vi "Floc Interface.vi"(8 "error in":errorcluster, 9 "ROI":T3, 10 "Interface inputs":T1={"Elevation of top of Field of View (cm)"=10.0, "Field of View Height (cm)"=-0.1, "Smooth Length (cm)"=5.0, "Min derivative magnitude"=5.0, "Color Plane"=enum."Green"} {"Smooth Length (cm)" min=0.01 max=1000.0 step=0.1; "Field of View Height (cm)" min=0.1 max=1000.0 step=0.1}, 11 "Image":T2) -> (0 "error out":errorcluster, 1 "max value":dbl, 2 "Interface elevation":dbl, 4 "min value":dbl)   [LabVIEW 2015, in "Camera SubVIs.lvlib"]
uses:
  Camera SubVIs.lvlib
  <vilib>/vision/Image Controls.llb/IMAQ Image.ctl
  Interface Inputs.ctl
  <vilib>/Analysis/baseanly.llb/Mean (DBL).vi
  <vilib>/Analysis/NI_AALBase.lvlib
  <vilib>/Analysis/NI_AALPro.lvlib
  <vilib>/vision/NI_Vision_Development_Module.lvlib
  <resource>/objmgr/IMAQImage.rc
panel:
  out "error out 2":errorcluster
  out "ROI Out":T2(plugin-control)
  out "min index":i32
  out "max index":i32
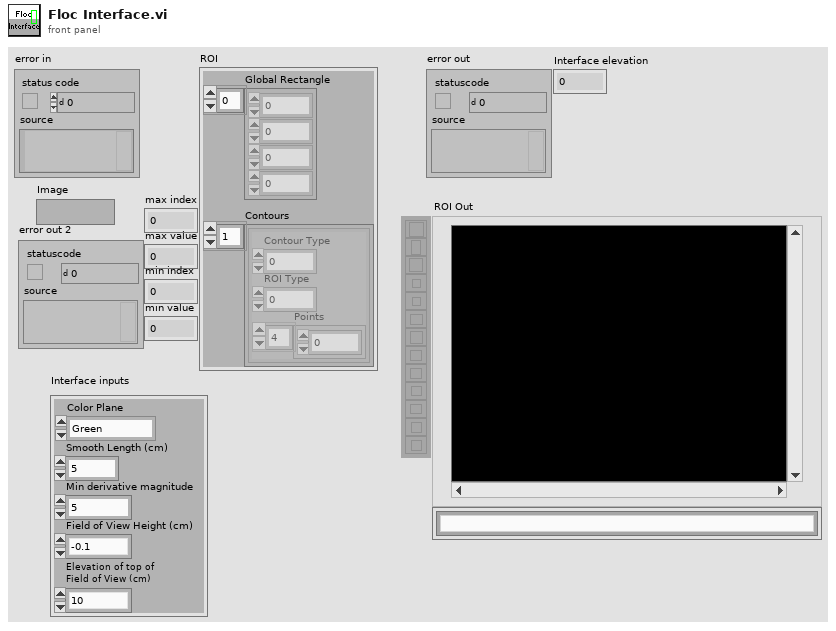
[diagram p1: front panel]
types:
  T1 = typedef "Camera SubVIs.lvlib/Interface Inputs.ctl" = cluster{"Elevation of top of Field of View (cm)":dbl, "Field of View Height (cm)":dbl, "Smooth Length (cm)":dbl, "Min derivative magnitude":dbl, "Color Plane":enum16{"Red", "Green", "Blue", "Combined"}}
  T2 = typedef "IMAQ Image.ctl" = refnum<image>
  T3 = cluster{"Global Rectangle":i32[], "Contours":cluster{"Contour Type":u32, "ROI Type":u32, "Points":i32[]}[]}
  T4 = typedef "Image Type" = u32
  T5 = cluster{"Global Rectangle[0]":i32, "Global Rectangle[1]":i32, "Global Rectangle[2]":i32, "Global Rectangle[3]":i32}
  T6 = cluster{"Red (or Hue) value":u8, "Green (or Sat) value":u8, "Blue (or Light or Val) value":u8}[][]
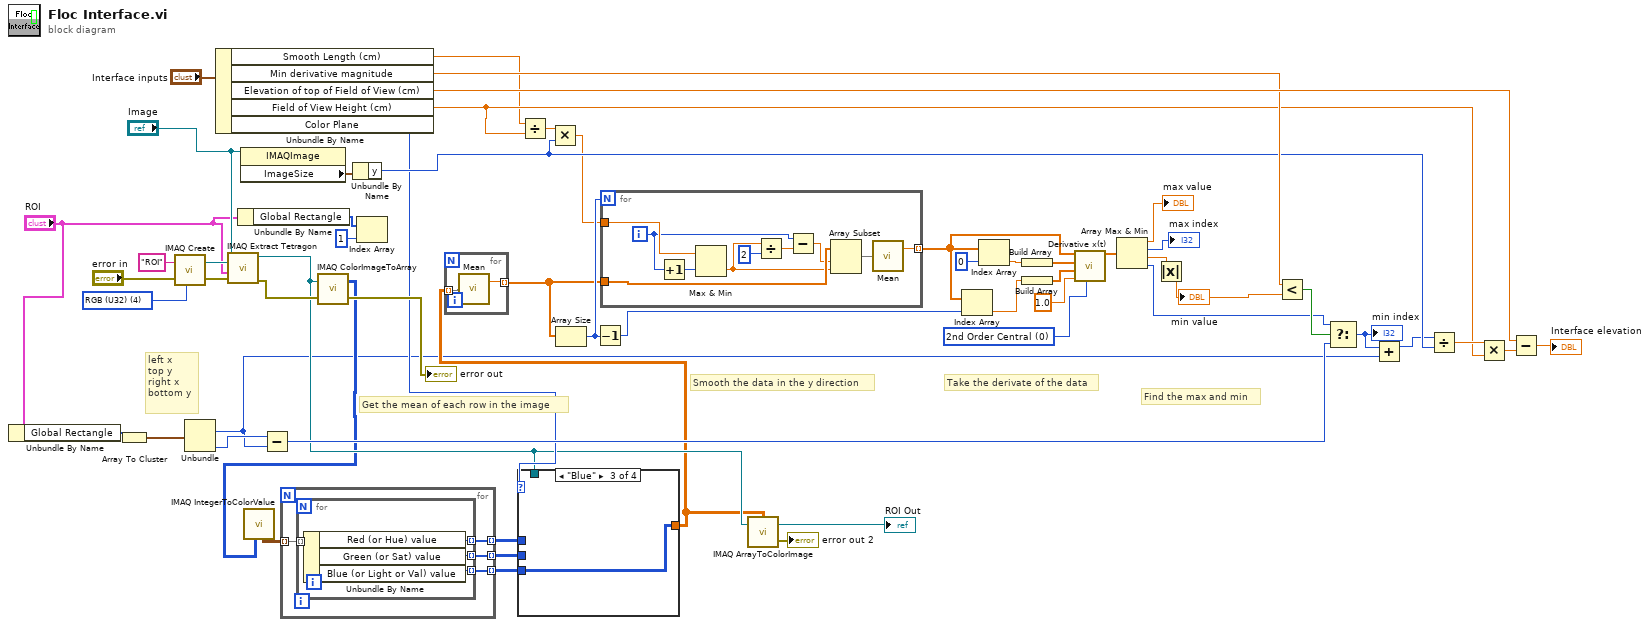
[diagram p0: block diagram]
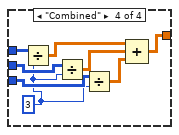
[diagram p4: hidden frame]
diagram:
  w43 = T4 4 items=["Grayscale (U8)", "Grayscale (I16)", "Grayscale (SGL)", "Complex (CSG)", "RGB (U32)", "HSL (U32)", "RGB (U64)", "Grayscale (U16)"] ("Image Type")
  w45 = u16 0 items=["2nd Order Central", "4th Order Central", "Forward", "Backward"] ("method")
  # "left x\ntop y\nright x\nbottom y"
  # "Find the max and min"
  # "Take the derivate of the data"
  # "Smooth the data in the y direction"
  # "Get the mean of each row in the image"
  n1 = Unbundle By Name("ROI") -> ("Global Rectangle"=w35:i32[])
  n2 = Array To Cluster(array=w35) -> (cluster=w34:T5)
  n3 = call "IMAQ Create"("Image Name"="ROI", "Image Type"=w43, "error in (no error)"="error in") -> ("New Image"=w40:T2, "error out"=w41:errorcluster)  [unwired: 1 in, 1 out]
  n4 = Unbundle(w34) -> ("Global Rectangle[1]"=w1:i32, "Global Rectangle[3]"=w33:i32)  [unwired: 2 out]
  n5 = Unbundle By Name("Interface inputs") -> ("Smooth Length (cm)"=w22:dbl, "Min derivative magnitude"=w25:dbl, "Elevation of top of Field of View (cm)"=w27:dbl, "Field of View Height (cm)"=w23:dbl, "Color Plane"=w17:enum16{"Red", "Green", "Blue", "Combined"})
  n6 = call-poly "IMAQ Extract Tetragon"("error in (no error)"=w41, "ROI Descriptor"="ROI", "Image Dst"=w40, "Image Src"="Image") -> ("error out"=w18:errorcluster, "Image Dst Out"=w14:T2)  [unwired: 6 in]
  n7 = Unbundle By Name("ROI") -> ("Global Rectangle"=w4:i32[])
  n8 = property class="IMAQImage"(reference="Image") -> ("ImageSize"=w6:cluster{"x":i32, "y":i32})  [unwired: 1 in, 2 out]
  n9 = Subtract(x=w33, y=w1) -> (x-y=w32:i32)
  n10 = call "IMAQ ColorImageToArray"("Image"=w14, "error in (no error)"=w18) -> ("Image Pixels (U32)"=w9:u32[][], "error out"=→"error out":errorcluster)  [unwired: 2 in, 1 out]
  n11 = call "IMAQ IntegerToColorValue"("2D U32 array"=w9) -> ("2D Color value array"=w13:T6)  [unwired: 4 in, 3 out]
  n12 = for {
    tunnel: w13 -> [w62] mode=indexing
    tunnel: [w61] -> w12 mode=indexing
    tunnel: [w60] -> w11 mode=indexing
    tunnel: [w59] -> w10 mode=indexing
    n13 = for {
      tunnel: w62 -> [w66] mode=indexing
      tunnel: [w65] -> w61 mode=indexing
      tunnel: [w64] -> w60 mode=indexing
      tunnel: [w63] -> w59 mode=indexing
      n14 = Unbundle By Name(w66) -> ("Red (or Hue) value"=w65:u8, "Green (or Sat) value"=w64:u8, "Blue (or Light or Val) value"=w63:u8)
    }
  }
  n15 = Unbundle By Name(w6) -> ("y"=w20:i32)
  n16 = Index Array(array=w4, index=1) -> ()  [unwired: 1 out]
  n17 = case shown="\"Blue\"" w17 {
    tunnel: [w67 w68 w69 w70] -> w8
    tunnel: w14 -> [_ _ _ _]
    tunnel: w12 -> [w67 _ _ w77]
    tunnel: w11 -> [_ w68 _ w76]
    tunnel: w10 -> [_ _ w69 w75]
    frame "Red", Default {
    }
    frame "Green" {
    }
    frame "Blue" {
    }
    frame "Combined" {
      w74 = 3
      n18 = Divide(x=w77, y=w74) -> (x/y=w73:dbl[][])
      n19 = Divide(x=w76, y=w74) -> (x/y=w72:dbl[][])
      n20 = Divide(x=w75, y=w74) -> (x/y=w71:dbl[][])
      n21 = Compound Arithmetic op=ADD(w73, w72, w71) -> (w70:dbl[][])
    }
  }
  n22 = for {
    tunnel: w8 -> [w79] mode=indexing
    tunnel: [w78] -> w7 mode=indexing
    n23 = call-poly <vilib>:"Mean.vi"("X"=w79) -> ("mean"=w78:dbl)  [unwired: 1 out]
  }
  n24 = Divide(x=w22, y=w23) -> (x/y=w21:dbl)
  n25 = Multiply(x=w21, y=w20) -> (x*y=w19:dbl)
  n26 = Array Size(array=w7) -> (size(s)=w52:i32)
  n27 = Decrement(x=w52) -> (x-1=w49:i32)
  n28 = for {
    N: w52 -> [_]
    tunnel: w7 -> [w89]
    tunnel: w19 -> [w86]
    tunnel: [w87] -> w51 mode=indexing
    i -> [w82]
    n29 = Increment(x=w82) -> (x+1=w85:i32)
    n30 = Max & Min(x=w86, y=w85) -> (min(x,y)=w84:dbl)  [unwired: 1 out]
    n31 = Divide(x=w84, y=2) -> (x/y=w80:dbl)
    n32 = Subtract(x=w82, y=w80) -> (x-y=w81:dbl)
    n33 = Array Subset(array=w89, index=w81, length=w84) -> (w88:dbl[])
    n34 = call-poly <vilib>:"Mean.vi"("X"=w88) -> ("mean"=w87:dbl)  [unwired: 1 out]
  }
  n35 = call "IMAQ ArrayToColorImage"("Image Pixels (U32)"=w8, "Image"=w14) -> ("Image Out"=→"ROI Out":T2, "error out"=→"error out 2":errorcluster)  [unwired: 3 in]
  n36 = Index Array(array=w51, index=w49) -> (element=w53:dbl)
  n37 = Index Array(array=w51, index=0) -> (element=w55:dbl)
  n38 = Build Array(w55) -> (w54:dbl[])
  n39 = Build Array(w53) -> (w50:dbl[])
  n40 = call <vilib>:"Derivative x(t).vi"("method"=w45, "dt"=1.0, "Final Condition"=w50, "Initial Condition"=w54, "X"=w51) -> ("dX/dt"=w57:dbl[])  [unwired: 5 in, 1 out]
  n41 = Array Max & Min(array=w57) -> (max value=→"max value":dbl, max index (indices)=→"max index":i32, min value=w46:dbl, min index (indices)=w36:i32)
  n42 = Absolute Value(x=w46) -> (abs(x)=w38:dbl)
  "min value" <- w38
  n43 = Less?(x=w25, y=w38) -> (x < y?=w37:bool)
  n44 = Select(t=w36, s=w37, f=w32) -> (s? t:f=w29:i32)
  "min index" <- w29
  n45 = Add(x=w29, y=w1) -> (x+y=w2:i32)
  n46 = Divide(x=w2, y=w20) -> (x/y=w28:dbl)
  n47 = Multiply(x=w28, y=w23) -> (x*y=w26:dbl)
  n48 = Subtract(x=w27, y=w26) -> (x-y=→"Interface elevation":dbl)
